vi "FTW-CodeGen-Prototype.vi"(1 "ADAPT_Array":string[](array[string])) -> (0 "ADAPT_Shuffled Array":string[](array[string]))   [LabVIEW 2014, in "FTW-Array-Shuffle.xnode"]
uses:
  FTW-Array-Shuffle.xnode
panel:
  # "Inputs"
  # "Outputs"
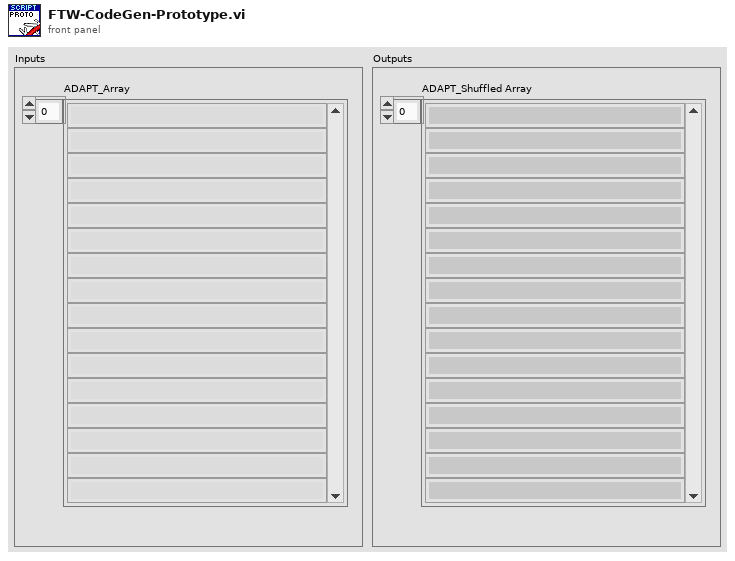
[diagram p1: front panel]
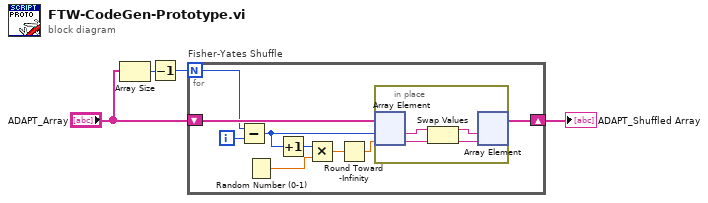
[diagram p0: block diagram]
diagram:
  n1 = Array Size(array="ADAPT_Array") -> (size(s)=w3:i32)
  n2 = Decrement(x=w3) -> (x-1=w4:i32)
  n3 = for "Fisher-Yates Shuffle" {
    N: w4 -> [w9]
    shift-right: [w12] -> w1
    shift-left: "ADAPT_Array" -> [w13]
    i -> [w8]
    n4 = Subtract(x=w9, y=w8) -> (x-y=w7:i32)
    n5 = Random Number (0-1)() -> (number: 0 to 1=w11:dbl)
    n6 = Increment(x=w7) -> (x+1=w6:i32)
    n7 = Multiply(x=w6, y=w11) -> (x*y=w10:dbl)
    n8 = Round Toward -Infinity(1:w10) -> (0:w5:dbl)
    n9 = in-place {
      n10 = in-place-array #1(w13, w7, w5) -> (w17:string, w15:string)
      n11 = Swap Values(12:w17, 14:w15) -> (1:w16:string, 3:w14:string)  [unwired: 1 in]
      n12 = in-place-array #1(w16, w14) -> (w12:string[])  [unwired: 2 out]
    }
  }
  "ADAPT_Shuffled Array" <- w1
